vi "log_to_csv.vi"(2 "error in":errorcluster, 3 "log file path":path=path "M:/ECE480/log.csv", 4 "channel 4 bit":string="11111001", 5 "channel 3 bit":string="11111001", 6 "channel 2 bit":string="11111001", 7 "channel 1 bit":string="11111001") -> (0 "appended array":u8[](array[numeric]), 1 "error out":errorcluster)   [LabVIEW 2021]
uses:
  <vilib>/Utility/file.llb/Write Delimited Spreadsheet (I64).vi
panel:
  out "output 4":u8
  out "output 3":u8
  out "output 2":u8
  out "output 1":u8
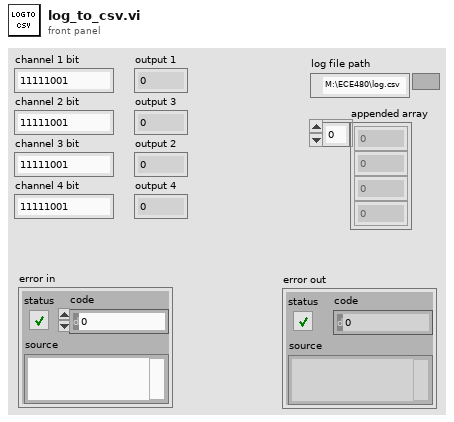
[diagram p1: front panel]
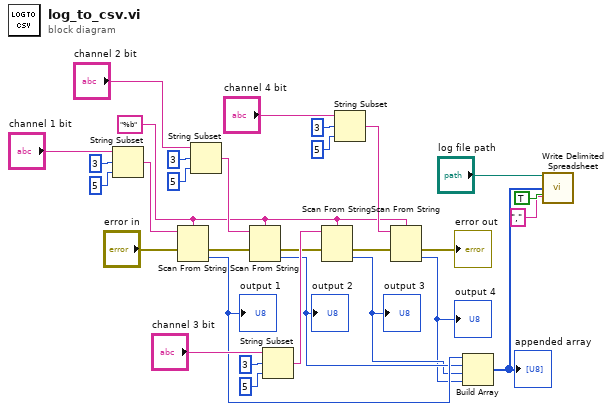
[diagram p0: block diagram]
diagram:
  w14 = "%b" ("format string")
  n1 = String Subset(string="channel 1 bit", offset (0)=3, length (rest)=5 ("length (rest)")) -> (substring=w18:string)
  n2 = Scan From String(format string=w14, input string=w18, error in="error in") -> (error out=w5:errorcluster, output 1=w13:u8)  [unwired: 2 in, 2 out]
  "output 1" <- w13
  n3 = String Subset(string="channel 2 bit", offset (0)=3, length (rest)=5 ("length (rest)")) -> (substring=w17:string)
  n4 = Scan From String(format string=w14, input string=w17, error in=w5) -> (error out=w4:errorcluster, output 1=w12:u8)  [unwired: 2 in, 2 out]
  "output 2" <- w12
  n5 = String Subset(string="channel 3 bit", offset (0)=3, length (rest)=5 ("length (rest)")) -> (substring=w16:string)
  n6 = Scan From String(format string=w14, input string=w16, error in=w4) -> (error out=w3:errorcluster, output 1=w11:u8)  [unwired: 2 in, 2 out]
  "output 3" <- w11
  n7 = String Subset(string="channel 4 bit", offset (0)=3, length (rest)=5 ("length (rest)")) -> (substring=w15:string)
  n8 = Scan From String(format string=w14, input string=w15, error in=w3) -> (error out=→"error out":errorcluster, output 1=w10:u8)  [unwired: 2 in, 2 out]
  "output 4" <- w10
  n9 = Build Array(w13, w12, w11, w10) -> (w1:u8[])
  "appended array" <- w1
  n10 = call-poly <vilib>:"Write Delimited Spreadsheet.vi"("file path (dialog if empty)"="log file path", "1D data"=w1, "append to file? (new file:F)"=TRUE, "delimiter (\\t)"="," ("delimiter (\\t)")) -> ()  [unwired: 10 in, 2 out]
